vi "Mixed graph przypisanie osi.vi"(7 "Wvm Rer in":refnum<vi>, 8 "error in (no error)":errorcluster, 11 "Data in":T1) -> (0 "error out":errorcluster, 2 "Przebiegi Wfm":waveform(dbl)[](array[waveform]), 3 "Data out":T1)   [LabVIEW 2013]
doc: "Use this template to build a VI to use as a subVI."
uses:
  Kontrolki/Przetwarzanie/Kanaly.ctl
  Kontrolki/GUI/Przypisanie osi Y.ctl
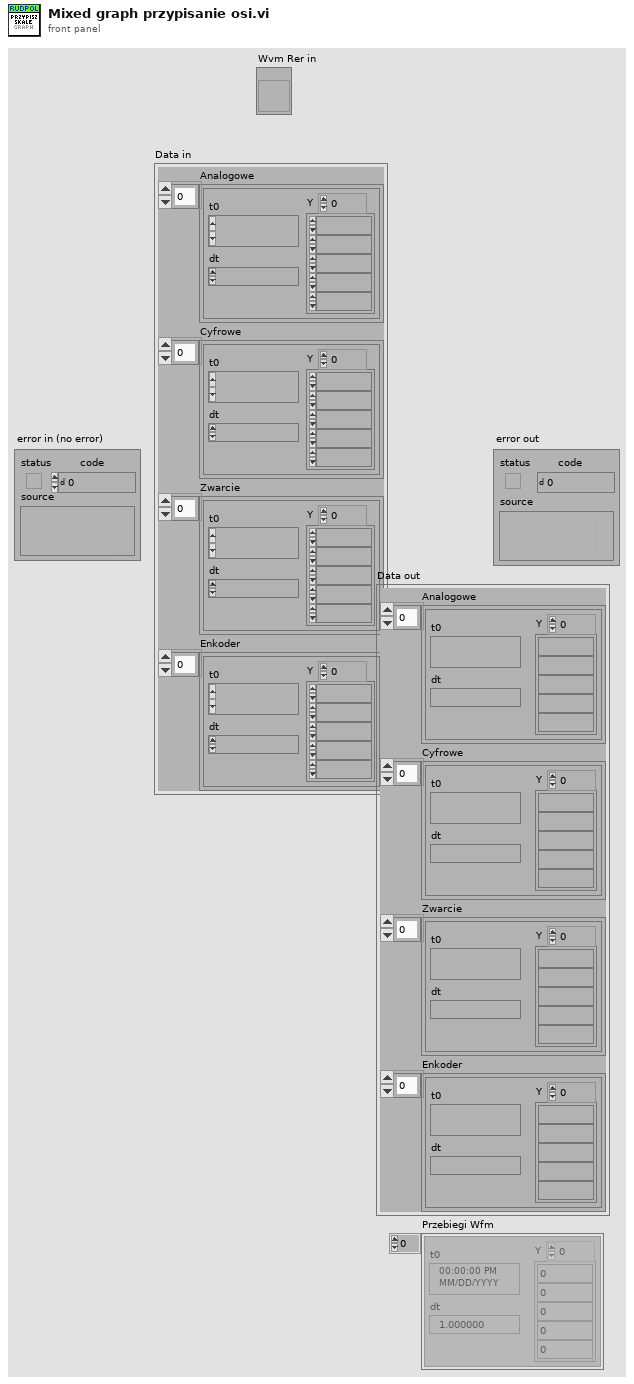
[diagram p1: front panel]
types:
  T1 = typedef "Kanaly.ctl" = cluster{"Analogowe":waveform(dbl)[], "Cyfrowe":waveform(dbl)[], "Zwarcie":waveform(dbl)[], "Enkoder":waveform(dbl)[]}
  T2 = typedef "Przypisanie osi Y.ctl" = enum16{"Enkoder", "Predkosc", "Przyspieszenie", "Analog 1", "Analog 2", "Znacznik"}
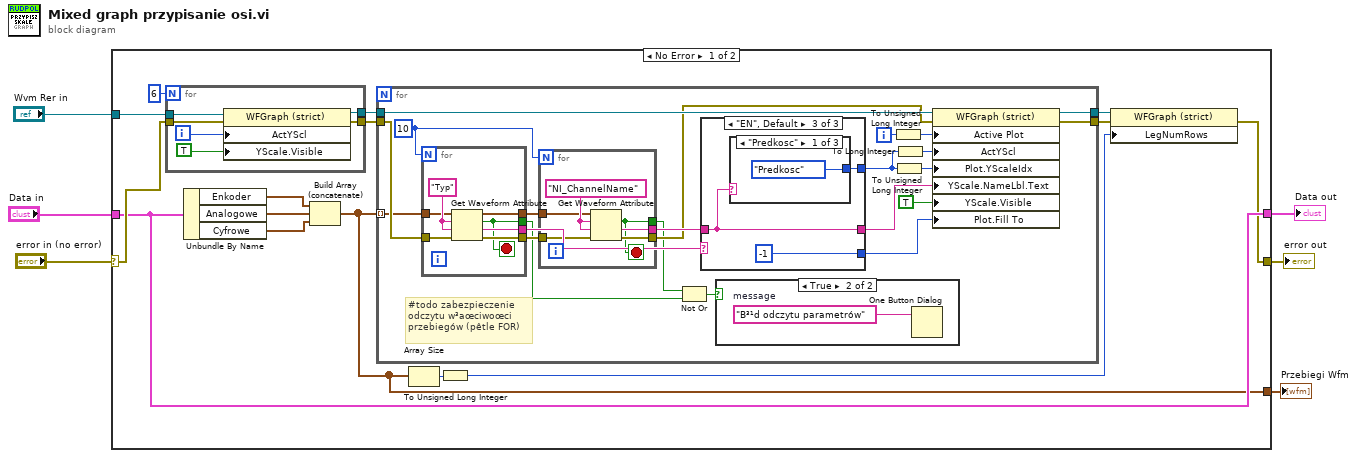
[diagram p0: block diagram]
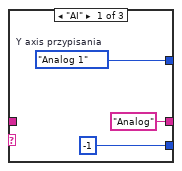
[diagram p3: hidden frame]
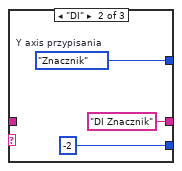
[diagram p4: hidden frame]
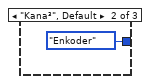
[diagram p5: hidden frame]
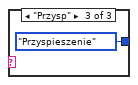
[diagram p6: hidden frame]
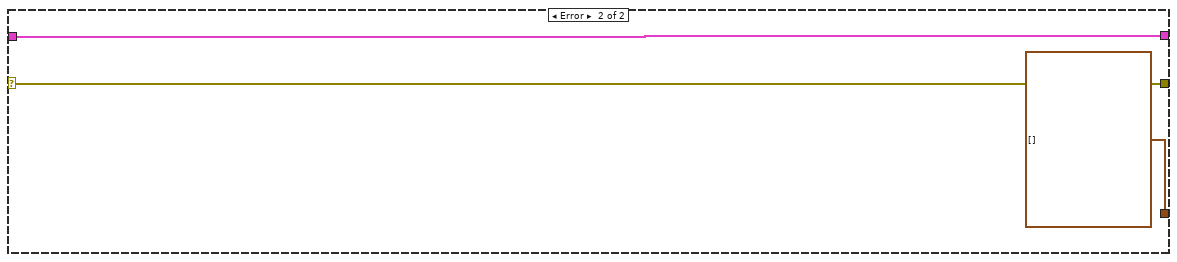
[diagram p7: hidden frame]
diagram:
  n1 = case shown="No Error" "error in (no error)" {
    selector: "error in (no error)" -> [w21 w78]
    tunnel: [w10 w78] -> w5
    tunnel: "Data in" -> [w16 w77]
    tunnel: [w16 w77] -> w2
    tunnel: "Wvm Rer in" -> [w20 _]
    tunnel: [w7 waveform(dbl)[] []] -> w1
    frame No Error {
      n2 = for {
        N: 6 -> [_]
        tunnel: w21 -> [w26]
        tunnel: w20 -> [w27]
        tunnel: [w23] -> w17
        tunnel: [w22] -> w18
        i -> [w25]
        n3 = property class="WFGraph (strict)"(reference=w27, error in=w26, "ActYScl"=w25, "YScale.Visible"=TRUE ("Y Scale.Visible")) -> (reference out=w22:refnum<vi>, error out=w23:errorcluster)
      }
      n4 = Unbundle By Name(w16) -> ("Enkoder"=w15:waveform(dbl)[], "Analogowe"=w14:waveform(dbl)[], "Cyfrowe"=w13:waveform(dbl)[])
      n5 = Build Array (concatenate)(w15, w14, w13) -> (w7:waveform(dbl)[])
      n6 = for {
        tunnel: w18 -> [w46]
        tunnel: w17 -> [w47]
        tunnel: [w35] -> w11
        tunnel: w7 -> [w34] mode=indexing
        tunnel: [w33] -> w9
        i -> [w49]
        w31 = 10
        # "#todo zabezpieczenie\nodczytu w³aœciwoœci\nprzebiegów (pêtle FOR)"
        n7 = for {
          N: w31 -> [_]
          tunnel: w47 -> [w62]
          tunnel: [w61] -> w42
          tunnel: [w60] -> w41
          tunnel: w34 -> [w59]
          tunnel: [w58] -> w32
          tunnel: [w57] -> w29
          stop <- w57 stop-if-true
          w63 = "Typ"
          n8 = Get Waveform Attribute(4:w62, 5:w63, 6:w63, 7:w59) -> (0:w60:errorcluster, 1:w58:string, 2:w57:bool, 3:w61:waveform(dbl))
        }
        n9 = for {
          N: w31 -> [_]
          tunnel: w42 -> [w55]
          tunnel: w41 -> [w54]
          tunnel: [w53] -> w40
          tunnel: [w52] -> w36
          tunnel: [w51] -> w30
          stop <- w51 stop-if-true
          w56 = "NI_ChannelName"
          n10 = Get Waveform Attribute(4:w54, 5:w56, 6:w56, 7:w55) -> (0:w52:errorcluster, 1:w53:string, 2:w51:bool)  [unwired: 1 out]
        }
        n11 = Not Or(1:w29, 2:w30) -> (0:w28:bool)
        n12 = case shown="\"EN\", Default" w32 {
          tunnel: [i16 -1 ("Plot.Fill To") i16 -2 ("Plot.Fill To") i16 -1 ("Plot.Fill To")] -> w44
          tunnel: ["Analog" "DI Znacznik" w71] -> w43
          tunnel: w40 -> [_ _ w71]
          tunnel: [w65 w68 w70] -> w37
          frame "AI" {
            w65 = Przypisanie_osi_Y."Analog 1"  # Y axis przypisania
          }
          frame "DI" {
            w68 = Przypisanie_osi_Y."Znacznik"  # Y axis przypisania
          }
          frame "EN", Default {
            n13 = case shown="\"Predkosc\"" w71 {
              tunnel: [Przypisanie_osi_Y."Predkosc" ("Y axis przypisania") Przypisanie_osi_Y."Enkoder" ("Y axis przypisania") Przypisanie_osi_Y."Przyspieszenie" ("Y axis przypisania")] -> w70
              frame "Predkosc" {
              }
              frame "Kana³", Default {
              }
              frame "Przysp" {
              }
            }
          }
        }
        n14 = case shown="True" w28 {
          frame False {
          }
          frame True {
            w50 = "B³¹d odczytu parametrów"  # message
            n15 = One Button Dialog(message=w50) -> ()  [unwired: 1 in, 1 out]
          }
        }
        n16 = To Unsigned Long Integer(number=w49) -> (unsigned 32bit integer=w48:u32)
        n17 = To Unsigned Long Integer(number=w37) -> (unsigned 32bit integer=w39:u32)
        n18 = To Long Integer(number=w37) -> (32bit integer=w38:i32)
        n19 = property class="WFGraph (strict)"(reference=w46, error in=w36, "Active Plot"=w48, "ActYScl"=w38, "Plot.YScaleIdx"=w39, "YScale.NameLbl.Text"=w43, "YScale.Visible"=TRUE ("Y Scale.Visible"), "Plot.Fill To"=w44) -> (reference out=w33:refnum<vi>, error out=w35:errorcluster)
      }
      n20 = Array Size(array=w7) -> (size(s)=w12:i32)
      n21 = To Unsigned Long Integer(number=w12) -> (unsigned 32bit integer=w8:u32)
      n22 = property on="Property Node" class="WFGraph (strict)"(reference=w9, error in=w11, "LegNumRows"=w8) -> (error out=w10:errorcluster)  [unwired: 1 out]
    }
    frame Error {
    }
  }
  "error out" <- w5
  "Data out" <- w2
  "Przebiegi Wfm" <- w1
